vi "slow_control_alpha_06.vi"() -> ()   [LabVIEW 2018]
uses:
  <instrlib>/Lake Shore 335/Lake Shore 335.lvlib
  <instrlib>/CAEN PSM/CAEN PSM.lvlib
panel:
  in  "Cycles to execute":dbl=5.0 format="%#_13g"
  out "Moving average Det. P":dbl
  in  "N samples":i32=20
  in  "Allows tabs on \nfront panel":T1(tab)
  in  "Heater range":u16(ring) items=["Off", "Low (On)", "Medium", "High"]
  in  "Setpoint (°C)":dbl=-100.0 format="%.1f"
  in  "PID settings":cluster{"P":dbl, "I":dbl, "D":dbl}={"P"=50.0, "I"=20.0, "D"=120.0}
  in  "COM-port NI-box":refnum<visa-resource-name>
  in  "COM-port LakeShore":refnum<visa-resource-name>
  in  "ID Query":bool=TRUE
  in  "COM-port CAEN 1":refnum<visa-resource-name>
  in  "COM-port CAEN 2":refnum<visa-resource-name>
  in  "Sensor 2 Offset":dbl=1.0 format="%#_13g"
  in  "Sensor 2 Mult. Factor":dbl=25.0 format="%#_13g"
  in  "Sensor 1 Offset":dbl=0.44736 format="%#_13g"
  in  "Sensor 1 Mult. Factor":dbl=25.0 format="%#_13g"
  in  "Sensor 3 Offset":dbl=1.0 format="%#_13g"
  in  "Sensor 3 Mult. Factor":dbl=50.0 format="%#_13g"
  in  "Sensor 4 Offset":dbl=1.0 format="%#_13g"
  in  "Sensor 4 Mult. Factor":dbl=10.0 format="%#_13g"
  in  "Ignore Initialization Errors":bool caption="Ignore init. errors?"
  out "LakeShore status":bool
  out "NI-box status":bool
  out "CAEN 1 status":bool
  out "CAEN 2 status":bool
  out "Initialization status":bool
  out "Heater power (%)":cluster{timestamp[], dbl[]}[](graph)
  out "Flow (SLPM)":cluster{timestamp[], dbl[]}[](graph)
  out "Pressure":cluster{timestamp[], dbl[]}[](graph)
  out "Phase Diagram":cluster{"X":dbl, "Y":dbl}[](graph)
  in  "Temp. Channel selector":string(combo)="Average 15 to 20"
  out "Temperature":cluster{timestamp[], dbl[]}[](graph)
  in  "N samples":i32=30
  out "Average Flow (SLPM)":dbl caption="Average Flow (SLPM), of"
  in  "Pause?":bool
  out "Integrated Flow (SL)":dbl
  in  "Reset?":bool
  out "Coldhead":dbl
  out "Heater":dbl
  out "Temp. 1":dbl
  out "Temp. 2":dbl
  out "Temp. 3":dbl
  out "Temp. 4":dbl
  out "Temp. 5":dbl
  out "Temp. 6":dbl
  out "Temp. 7":dbl
  out "Temp. 8":dbl
  out "Temp. 9":dbl
  out "Temp. 10":dbl
  out "Temp. 11":dbl
  out "Temp. 12":dbl
  out "Temp. 13":dbl
  out "Temp. 14":dbl
  out "Temp. 15":dbl
  out "Temp. 16":dbl
  out "Temp. 17":dbl
  out "Temp. 18":dbl
  out "Temp. 19":dbl
  out "Temp. 20":dbl
  out "1 to 4":dbl[](array[numeric])
  out "5 to 8":dbl[](array[numeric])
  out "9 to 12":dbl[](array[numeric])
  out "13 to 16":dbl[](array[numeric])
  out "17 to 20":dbl[](array[numeric])
  out "Temp A":dbl
  out "Temp B":dbl
  in  "Temperature Channel selector":string(combo)="Average 15 to 20"
  out "Historical Large Phase Diagram":cluster{dbl[], dbl[]}[](graph)
  out "Large Phase Diagram":cluster{"X":dbl, "Y":dbl}[](graph)
  in  "Temperature Channel selector":string(combo)="Average 15 to 20"
  in  "Set to zero":bool
  out "Bottom gate":dbl(knob) scale=0.0..-3000.0
  out "Top gate":dbl(knob) scale=0.0..3000.0
  in  "Apply Voltage":bool
  in  "VSet (V)":dbl[](array[numeric])
  in  "IMax (uA)":dbl[](array[numeric])
  in  "VMax (V)":dbl[](array[numeric])
  out "Cathode":dbl(knob) scale=0.0..-5000.0
  out "Anode":dbl(knob) scale=0.0..4000.0
  out "PMT 2":dbl(knob) scale=0.0..1000.0
  out "PMT 1":dbl(knob) scale=1.0..1000.0
  out "Vmon (V)":dbl[](array[numeric])
  out "IMon (uA)":dbl[](array[numeric])
  out "Read V = 0":i32
  in  "Read V every N cycles":i16=120
  in  "Reset anode":bool
  in  "Kill every Y minutes":i32=10
  in  "Keep off for X seconds":i32=10
  out "?":bool
  out "Killed":bool
  out "Restarted":bool
  out "Anode times":dbl[](array[numeric]) format="%_12f"
  in  "Kill voltage":bool
  in  "stop":bool
  out "Voltages":dbl[](array[numeric])
  out "Started up?":bool
  out "TOBA appended":dbl[][](array[numeric])
  in  "Read T every N cycles":i32=2
  out "Time until next cycle":dbl format="%.3g"
  in  "Time per cycle (s)":i32=2 caption="Time Target (s)"
  in  "input cluster":errorcluster
  # "<- Proof of concept for New/Old T + New P"
  # "PMT 1"
  # "PMT 2"
  # "Anode"
  # "Cathode"
  # "Top gate"
  # "Bottom gate"
  # "Pressure correction settings"
  # "Connection settings"
  # "Lakeshore settings"
  # "Gain (P) (XX.X)"
  # "Reset (I) (XX.X)"
  # "Rate (D) (X.X%)"
  # "<- Change wiring,\nused for testing rn"
  # "Might need to split up NI-box com port.\nPreferable to task it with measuring T\nand P seperately.\nPerhaps need to set task per single channel."
  # "Alarm indicators"
  # "CAEN 1"
  # "Data"
  # "PMT 1"
  # "PMT 1"
  # "PMT 2"
  # "PMT 2"
  # "Anode"
  # "Anode"
  # "Cathode"
  # "Cathode"
  # "Top gate"
  # "Top gate"
  # "Bottom gate"
  # "Bottom gate"
  # "Settings"
  # "PMT 1"
  # "PMT 1"
  # "PMT 2"
  # "PMT 2"
  # "Anode"
  # "Anode"
  # "Cathode"
  # "Cathode"
  # "Top gate"
  # "Top gate"
  # "Bottom gate"
  # "Bottom gate"
  # "CAEN 2"
  # "PMT 1"
  # "PMT 2"
  # "Anode"
  # "seconds"
  # "Cathode"
  # "Needle gauges or other displays go here"
  # "Top gate"
  # "Bottom gate"
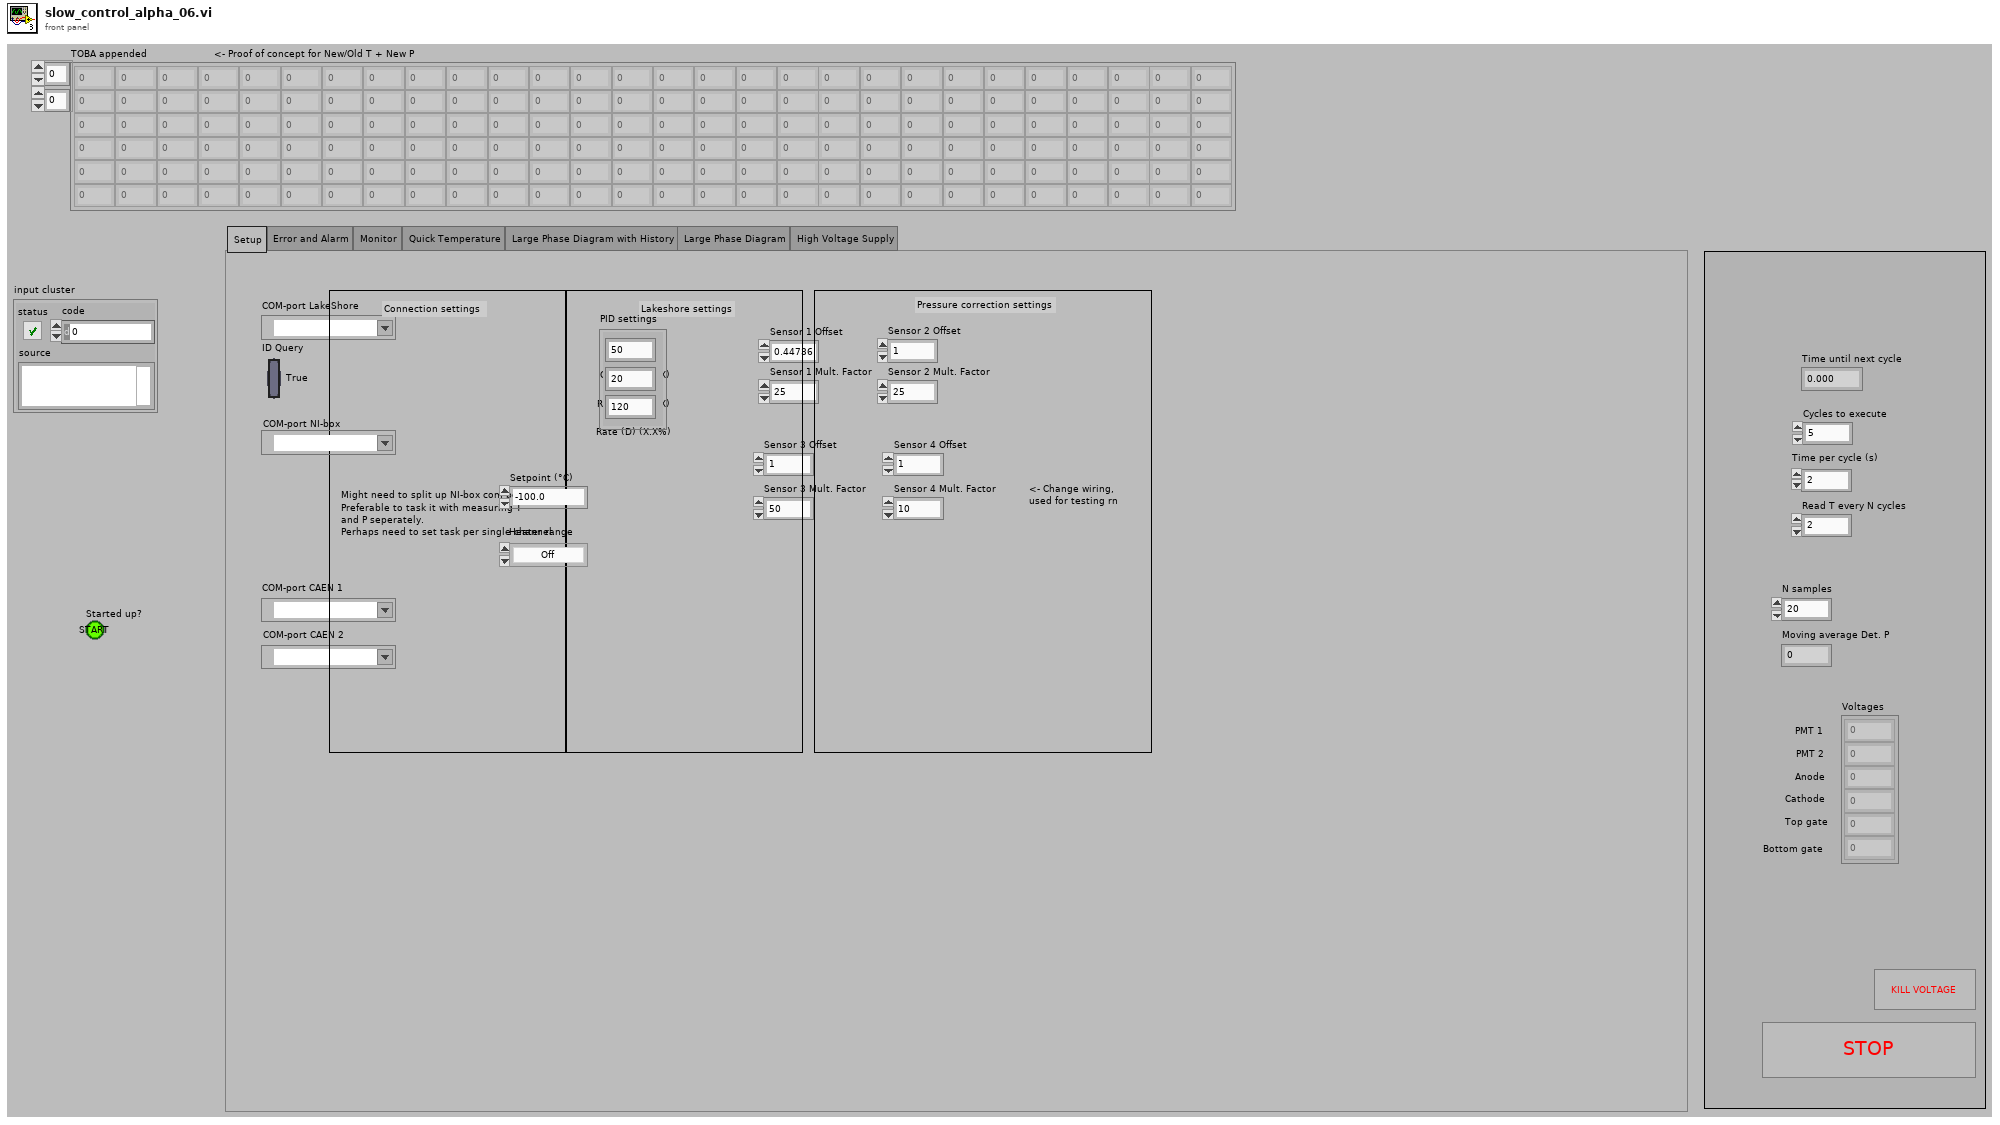
[diagram p1: front panel]
types:
  T1 = enum32{"Setup", "Error and Alarm", "Monitor", "Quick Temperature", "Large Phase Diagram with History", "Large Phase Diagram", "High Voltage Supply"}
  T2 = cluster{"Flow Control":u16, "Stop Bits":u16, "Data Bits":u16, "Parity":u16, "Baud Rate":u32}
  T3 = cluster{"VISA resource name out":refnum<visa-resource-name>, "error out":errorcluster}
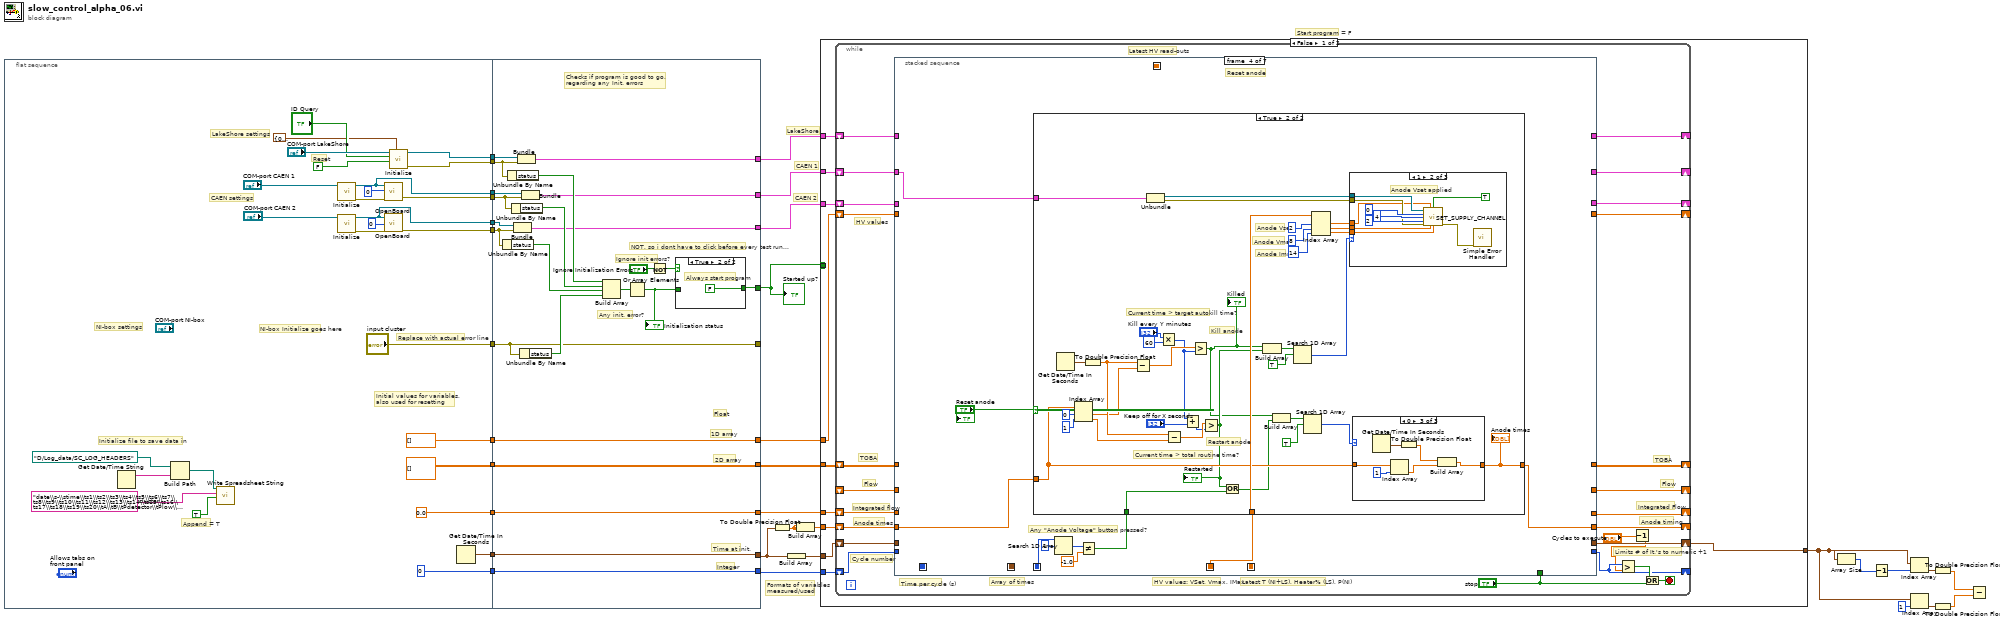
[diagram p0: block diagram]
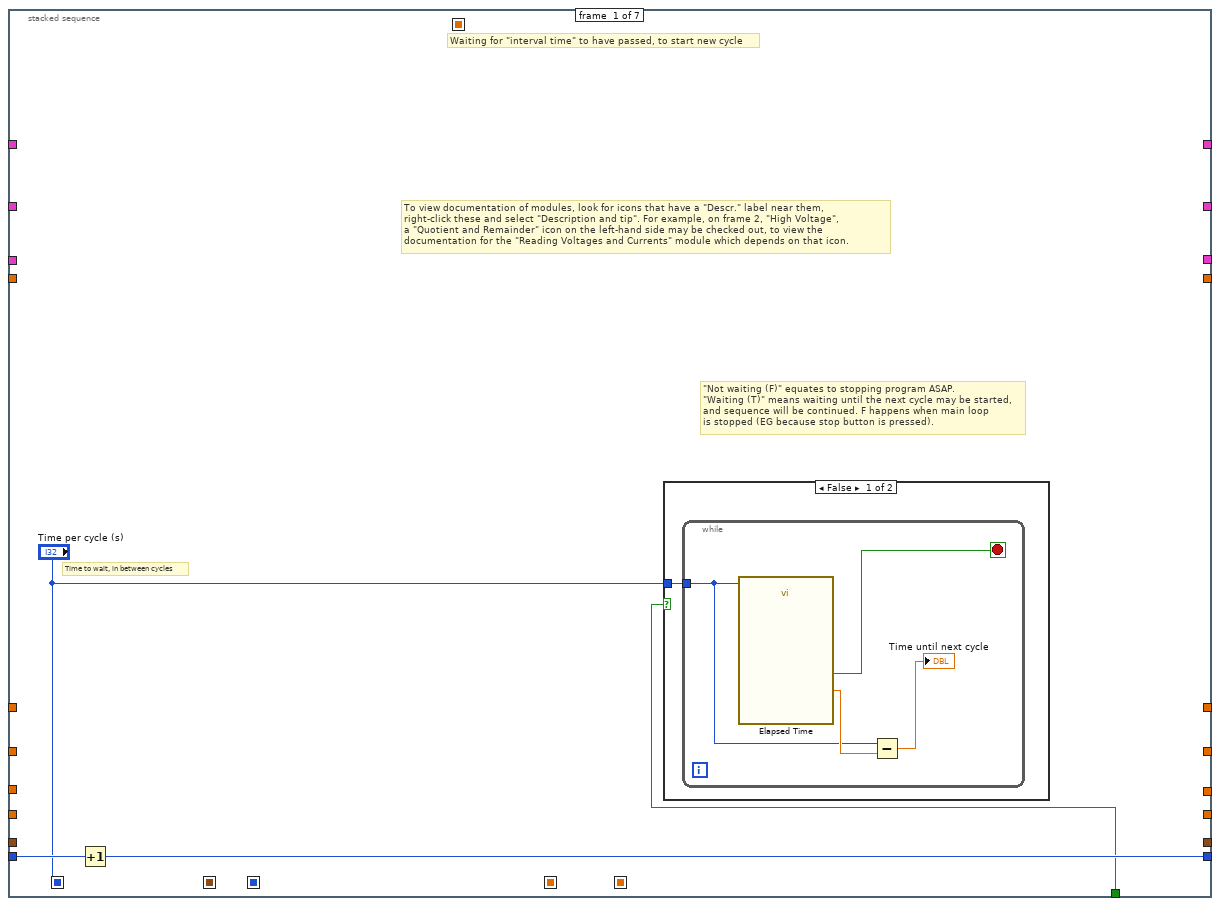
[diagram p2: hidden frame]
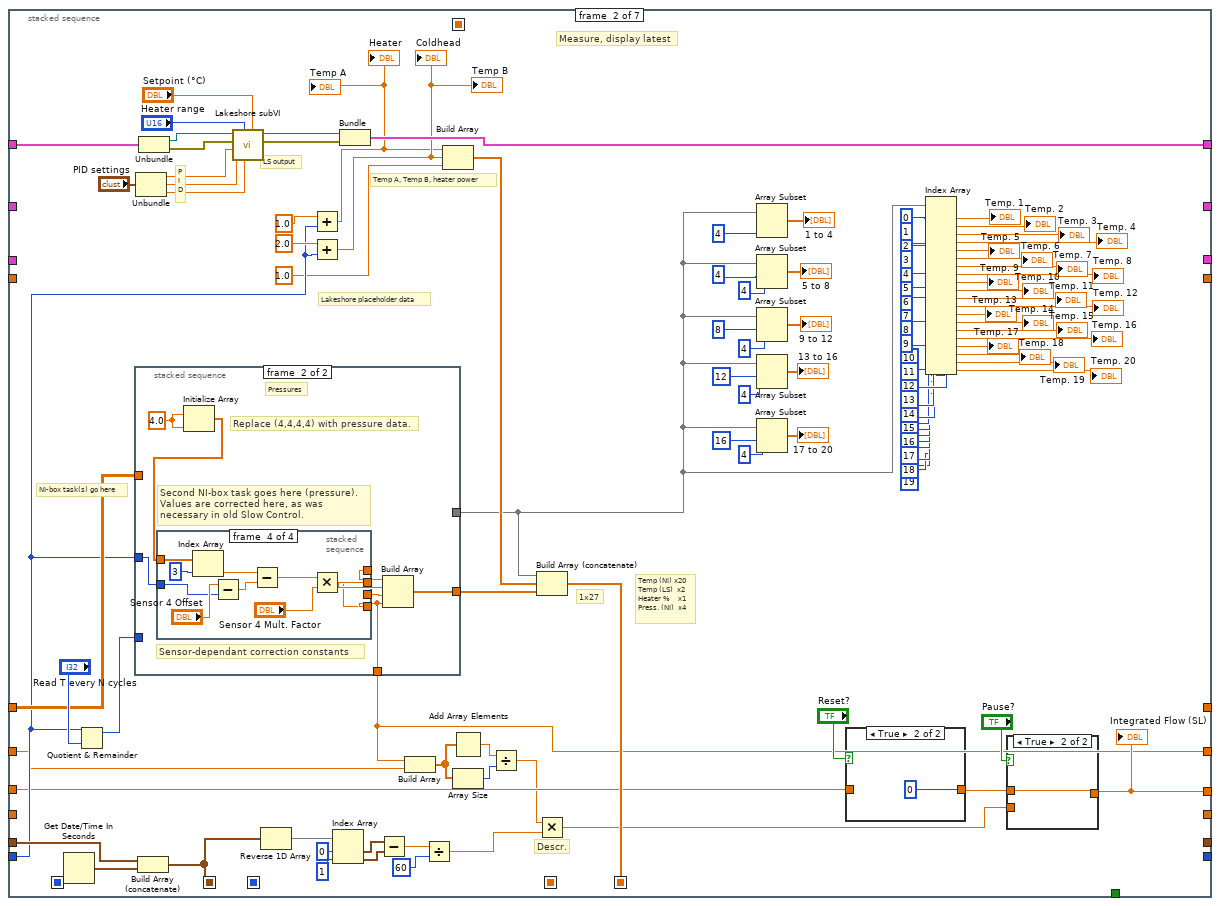
[diagram p4: hidden frame]
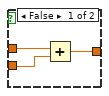
[diagram p6: hidden frame]
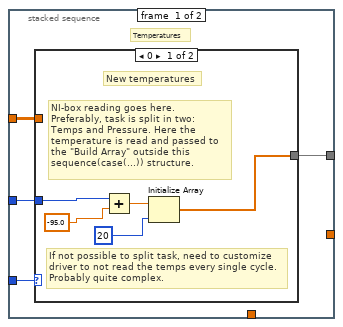
[diagram p7: hidden frame]
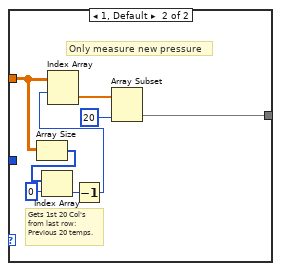
[diagram p8: hidden frame]
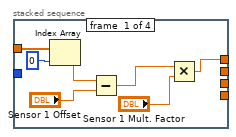
[diagram p9: hidden frame]
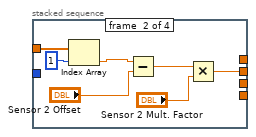
[diagram p10: hidden frame]
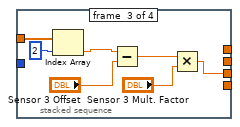
[diagram p11: hidden frame]
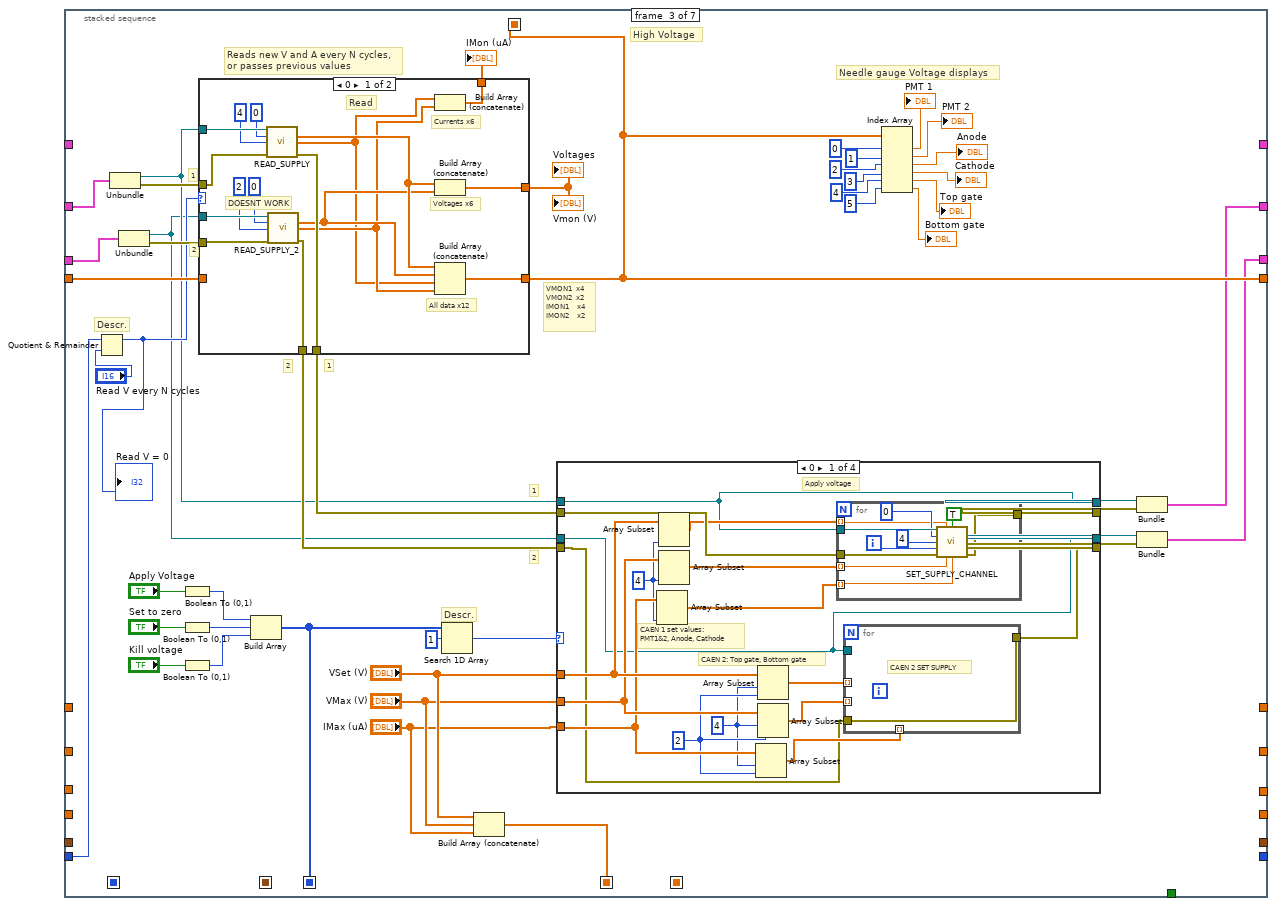
[diagram p12: hidden frame]
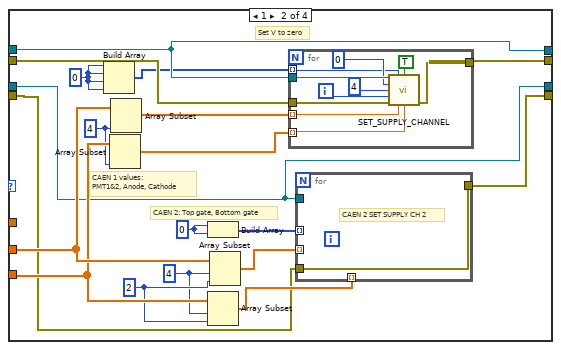
[diagram p13: hidden frame]
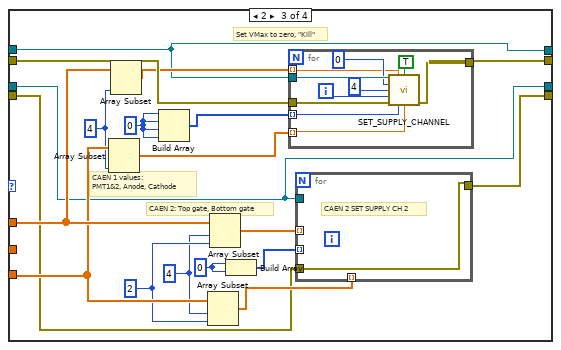
[diagram p14: hidden frame]
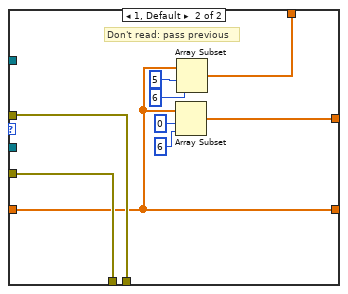
[diagram p16: hidden frame]
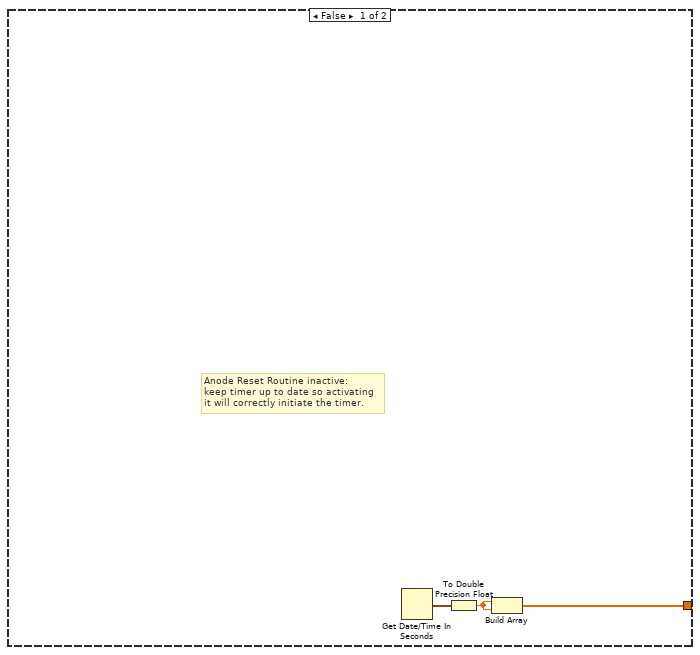
[diagram p17: hidden frame]
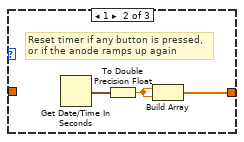
[diagram p19: hidden frame]
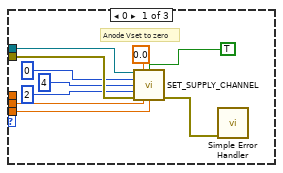
[diagram p20: hidden frame]
diagram:
  # "Start program = F"
  # "CAEN 2"
  # "CAEN 1"
  # "LakeShore"
  # "Formats of variables\nmeasured/used"
  n1 = flat-sequence {
    tunnel: [w56] -> w32
    tunnel: [w55] -> w31
    tunnel: [w51] -> w30
    tunnel: [w50] -> w29
    tunnel: ["input cluster"] -> w28
    tunnel: [0.0] -> w27
    tunnel: [dbl[] []] -> w26
    tunnel: [dbl[][] []] -> w25
    tunnel: [0] -> w24
    tunnel: [w38] -> w18
    tunnel: [w34] -> w8
    tunnel: [w33] -> w7
    tunnel: w32 -> [w72]
    tunnel: w31 -> [w71]
    tunnel: w30 -> [w69]
    tunnel: w29 -> [w68]
    tunnel: w28 -> [w73]
    tunnel: [w79] -> w5
    tunnel: [w77] -> w4
    tunnel: w27 -> [w77]
    tunnel: [w76] -> w23
    tunnel: w26 -> [w76]
    tunnel: [w75] -> w21
    tunnel: w25 -> [w75]
    tunnel: [w74] -> w22
    tunnel: w24 -> [w74]
    tunnel: [w73] -> _
    tunnel: [w70] -> w20
    tunnel: [w67] -> w19
    tunnel: [w64] -> w3
    tunnel: w18 -> [w64]
    tunnel: w8 -> [w62]
    tunnel: w7 -> [w61]
    tunnel: [w60] -> w6
    frame #0 {
      # "Append = T"
      # "Change to fit order of data in cluster"
      # "Initialize file to save data in"
      # "Initial values for variables,\nalso used for resetting"
      # "Replace with actual error line"
      # "NI-box Initialize goes here"
      # "NI-box settings"
      # "CAEN settings"
      # "Reset"
      # "LakeShore settings"
      n2 = Get Date/Time String() -> (date string=w41:string)  [unwired: 3 in, 1 out]
      n3 = Build Path(base path=path "D:/Log_data/SC_LOG_HEADERS", name or relative path=w41) -> (appended path=w44:path)
      n4 = call <vilib>:"Write Spreadsheet String.vi"("append to file? (new file:F)"=TRUE, "spreadsheet string"="date\\s-\\stime\\ts1\\ts2\\ts3\\ts4\\ts5\\ts6\\ts7\\ts8\\ts9\\ts10\\ts11\\ts12\\ts13\\ts14\\ts15\\ts16\\ts17\\ts18\\ts19\\ts20\\tA\\tB\\tPdetector\\tPlow\\tPhigh\\tFlow\\tHeater\\tSetpoint\\tCapacitance\\tTimestamp\\tInterval\\tLevel\\tV_PMT1\\tV_PMT2\\tV_Anode\\tV_cathode\\tI_PMT1\\tI_PMT2\\tI_Anode\\tI_cathode\\t\\r\\n", "file path (dialog if empty)"=w44) -> ()  [unwired: 7 in, 2 out]
      n5 = call <instrlib>:"Initialize.vi"("VISA resource name"="COM-port CAEN 1") -> ("error out"=w52:errorcluster, "VISA resource name out"=w51:refnum<visa-resource-name>)  [unwired: 9 in]
      n6 = call <instrlib>:"Initialize.vi"("VISA resource name"="COM-port CAEN 2") -> ("error out"=w35:errorcluster, "VISA resource name out"=w34:refnum<visa-resource-name>)  [unwired: 9 in]
      n7 = call <instrlib>:"OpenBoard.vi"("error in (no error)"=w52, "Board Address"=0, "VISA resource name"=w51) -> ("error out"=w50:errorcluster)  [unwired: 7 in, 1 out]
      n8 = call <instrlib>:"OpenBoard.vi"("error in (no error)"=w35, "Board Address"=u8 0, "VISA resource name"=w34) -> ("error out"=w33:errorcluster)  [unwired: 7 in, 1 out]
      n9 = call <instrlib>:"Initialize.vi"("Serial Configuration"=T2 {"Flow Control"=0, "Stop Bits"=10, "Data Bits"=7, "Parity"=1, "Baud Rate"=57600}, "Reset (True)"=FALSE ("Reset (LakeShore)"), "ID Query (True)"="ID Query", "VISA resource name"="COM-port LakeShore") -> ("error out"=w55:errorcluster, "VISA resource name out"=w56:refnum<visa-resource-name>)  [unwired: 6 in]
      n10 = Get Date/Time In Seconds() -> (seconds since 1Jan1904=w38:timestamp)
    }
    frame #1 {
      # "NOT, so i dont have to click before every test run..."
      # "Time at init."
      # "Integer"
      # "2D array"
      # "1D array"
      # "Float"
      # "Checks if program is good to go,\nregarding any Init. errors"
      # "Ignore init errors?"
      # "Any init. error?"
      n11 = Unbundle By Name(w61) -> ("status"=w63:bool)
      n12 = Unbundle By Name(w71) -> ("status"=w80:bool)
      n13 = Unbundle By Name(w68) -> ("status"=w82:bool)
      n14 = Bundle("VISA resource name out"=w62, "error out"=w61) -> (w60:T3)  [unwired: 1 in]
      n15 = Bundle("VISA resource name out"=w72, "error out"=w71) -> (w70:T3)  [unwired: 1 in]
      n16 = Unbundle By Name(w73) -> ("status"=w81:bool)
      n17 = Bundle("VISA resource name out"=w69, "error out"=w68) -> (w67:T3)  [unwired: 1 in]
      n18 = Build Array(w80, w82, w81, w63) -> (w83:bool[])
      n19 = Or Array Elements(Boolean array=w83) -> (logical OR=w78:bool)
      "Initialization status" <- w78
      n20 = Not(x="Ignore Initialization Errors") -> (.not. x?=w65:bool)
      n21 = case shown="True" w65 {
        tunnel: [w84 FALSE] -> w79
        tunnel: w78 -> [w84 _]
        frame False {
          # "Only start if no errors"
        }
        frame True {
          # "Always start program"
        }
      }
    }
  }
  n22 = To Double Precision Float(number=w3) -> (double precision float=w2:dbl)
  n23 = Build Array(w3) -> (w17:timestamp[])
  n24 = Build Array(w2, w2) -> (w1:dbl[])
  n25 = case shown="False" w5 {
    selector: w5 -> [_ w682]
    tunnel: [_ w682] -> _
    tunnel: w23 -> [w88 _]
    tunnel: w22 -> [w95 _]
    tunnel: w21 -> [w94 _]
    tunnel: w20 -> [w89 _]
    tunnel: w19 -> [w91 _]
    tunnel: w17 -> [w93 _]
    tunnel: [w92 timestamp[] []] -> w13
    tunnel: w6 -> [w90 _]
    tunnel: w4 -> [w87 _]
    tunnel: w1 -> [w86 _]
    frame False {
      n26 = while {
        shift-right: [w114] -> _
        shift-left: w95 -> [w120]
        shift-right: [w116] -> _
        shift-left: w94 -> [w105]
        shift-right: [w106] -> w92
        shift-left: w93 -> [w115]
        shift-right: [w108] -> _
        shift-left: w91 -> [w97]
        shift-right: [w110] -> _
        shift-left: w88 -> [w113]
        shift-right: [w107] -> _
        shift-left: w90 -> [w112]
        shift-right: [w109] -> _
        shift-left: w89 -> [w111]
        shift-right: [w104] -> _
        shift-left: w87 -> [w99]
        shift-right: [w101] -> _
        shift-left: _ -> [w100]
        shift-right: [w96] -> _
        shift-left: w86 -> [w98]
        stop <- w117 stop-if-true
        # "Anode timing"
        # "Anode times"
        # "Integrated flow"
        # "Flow"
        # "Flow"
        # "Integrated Flow"
        # "TOBA"
        # "Array of times"
        # "Latest HV read-outs"
        # "Time per cycle (s)"
        # "Cycle number"
        # "HV values: VSet, Vmax, IMax"
        # "HV values"
        # "TOBA"
        # "Latest T (NI+LS), Heater% (LS), P(NI)"
        # "Limits # of It.'s to numeric +1"
        n27 = stacked-sequence {
          seq-local: [_ w228 _ _ _ _ _] -> [_ _ _ _ w572 _ _]
          seq-local: [_ _ w294 _ _ _ _] -> [_ _ _ w460 _ _ _]
          seq-local: ["Time per cycle (s)" _ _ _ _ _ _] -> [_ _ _ _ _ _ _]
          seq-local: [_ _ w316 _ _ _ _] -> [_ _ _ _ _ _ _]
          seq-local: [_ w138 _ _ _ _ _] -> [_ _ _ _ w550 _ _]
          seq-local: [_ _ w293 _ _ _ _] -> [_ _ _ w465 _ _ _]
          tunnel: [w123 _ _ _ _ _ _] -> w114
          tunnel: "stop" -> [w122 _ _ _ _ _ _]
          tunnel: w120 -> [w124 w209 w331 _ _ _ _]
          tunnel: w105 -> [_ w229 _ _ w579 _ _]
          tunnel: [_ _ _ _ w571 _ _] -> w116
          tunnel: w115 -> [_ w215 _ _ _ _ _]
          tunnel: w97 -> [_ _ w338 w461 _ _ w678]
          tunnel: w113 -> [_ _ w336 _ _ _ _]
          tunnel: w112 -> [_ _ w335 _ _ _ w677]
          tunnel: w111 -> [_ w216 _ _ _ _ w675]
          tunnel: [_ w218 _ _ _ _ _] -> w109
          tunnel: [_ _ w316 _ _ _ _] -> w110
          tunnel: [_ _ w302 _ _ _ _] -> w108
          tunnel: [_ _ w299 _ _ _ _] -> w107
          tunnel: [_ _ _ _ w550 _ _] -> w106
          tunnel: w99 -> [_ w201 _ _ _ _ _]
          tunnel: [_ w202 _ _ _ _ _] -> w104
          tunnel: [_ w132 _ _ _ _ _] -> w101
          tunnel: w100 -> [_ w131 _ _ _ _ _]
          tunnel: w98 -> [_ _ _ w462 _ _ _]
          tunnel: [_ _ _ w458 _ _ _] -> w96
          frame #0 {
            # "To view documentation of modules, look for icons that have a \"Descr.\" label near them,\nright-click these and select \"Description and tip\". For example, on frame 2, \"High Voltage\",\na \"Quotient and Remainder\" icon on the left-hand side may be checked out, to view the\ndocumentation for the \"Reading Voltages and Currents\" module which depends on that icon."
            # "Time to wait, in between cycles"
            # "\"Not waiting (F)\" equates to stopping program ASAP.\n\"Waiting (T)\" means waiting until the next cycle may be started,\nand sequence will be continued. F happens when main loop \nis stopped (EG because stop button is pressed)."
            # "Waiting for \"interval time\" to have passed, to start new cycle"
            n28 = Increment(x=w124) -> (x+1=w123:i32)
            n29 = case shown="False" w122 {
              tunnel: "Time per cycle (s)" -> [w125 _]
              frame False {
                n30 = while {
                  tunnel: w125 -> [w127]
                  stop <- w129 stop-if-true
                  n31 = call "Elapsed Time"("Time Target (s)"=w127) -> ("Elapsed Time (s)"=w128:dbl, "Time has Elapsed"=w129:bool)  [unwired: 11 in, 6 out]
                  n32 = Subtract(x=w127, y=w128) -> (x-y=→"Time until next cycle":dbl)
                }
              }
              frame True {
              }
            }
          }
          frame #1 {
            # "1x27"
            # "Descr."
            # "LS output"
            # "Lakeshore placeholder data"
            # "Temp (NI) x20\nTemp (LS)  x2\nHeater %    x1\nPress. (NI)  x4"
            # "Temp A, Temp B, heater power"
            # "P\nI\nD"
            # "NI-box task(s) go here"
            # "Measure, display latest"
            n33 = Get Date/Time In Seconds() -> (seconds since 1Jan1904=w214:timestamp)
            n34 = Quotient & Remainder(x=w209, y="Read T every N cycles") -> (x-y*floor(x/y)=w230:i32)  [unwired: 1 out]
            n35 = stacked-sequence {
              tunnel: w230 -> [w241 _]
              tunnel: [w240 _] -> w136
              tunnel: [_ w259] -> w212
              tunnel: w229 -> [w239 _]
              tunnel: w209 -> [w238 w256]
              tunnel: [_ w255] -> w132
              frame #0 {
                # "Temperatures"
                n36 = case shown="0" w241 {
                  tunnel: w239 -> [_ w251]
                  tunnel: [w244 w247] -> w240
                  tunnel: w238 -> [w243 _]
                  frame 0 {
                    # "If not possible to split task, need to customize\ndriver to not read the temps every single cycle.\nProbably quite complex."
                    # "NI-box reading goes here.\nPreferably, task is split in two: \nTemps and Pressure. Here the \ntemperature is read and passed to \nthe \"Build Array\" outside this \nsequence(case(...)) structure."
                    # "New temperatures"
                    n37 = Add(x=w243, y=-95.0 ("element")) -> (x+y=w246:dbl)
                    n38 = Initialize Array(w246, 20) -> (w244:dbl[])
                  }
                  frame 1, Default {
                    # "Gets 1st 20 Col's\nfrom last row:\nPrevious 20 temps."
                    # "Only measure new pressure"
                    n39 = Array Size(array=w251) -> (size(s)=w253:i32[])
                    n40 = Index Array(array=w253, index=0) -> (element=w254:i32)
                    n41 = Decrement(x=w254) -> (x-1=w250:i32)
                    n42 = Index Array(array=w251, index (row)=w250) -> (element=w249:dbl[])  [unwired: 1 in]
                    n43 = Array Subset(array=w249, length=20) -> (w247:dbl[])  [unwired: 1 in]
                  }
                }
              }
              frame #1 {
                w258 = 4.0 ("element")
                # "Replace (4,4,4,4) with pressure data."
                # "Second NI-box task goes here (pressure).\nValues are corrected here, as was \nnecessary in old Slow Control."
                # "Sensor-dependant correction constants"
                # "Pressures"
                n44 = Initialize Array(w258, w258) -> (w257:dbl[])
                n45 = stacked-sequence {
                  tunnel: w257 -> [w264 w276 w283 w292]
                  tunnel: [w265 _ _ _] -> w262
                  tunnel: [_ w271 _ _] -> w261
                  tunnel: [_ _ w278 _] -> w260
                  tunnel: [_ _ _ w288] -> w255
                  tunnel: w256 -> [_ _ _ w284]
                  frame #0 {
                    n46 = Index Array(array=w264, index=0) -> (element=w263:dbl)
                    n47 = Subtract(x=w263, y="Sensor 1 Offset") -> (x-y=w267:dbl)
                    n48 = Multiply(x=w267, y="Sensor 1 Mult. Factor") -> (x*y=w265:dbl)
                  }
                  frame #1 {
                    n49 = Index Array(array=w276, index=1) -> (element=w270:dbl)
                    n50 = Subtract(x=w270, y="Sensor 2 Offset") -> (x-y=w273:dbl)
                    n51 = Multiply(x=w273, y="Sensor 2 Mult. Factor") -> (x*y=w271:dbl)
                  }
                  frame #2 {
                    n52 = Index Array(array=w283, index=2) -> (element=w277:dbl)
                    n53 = Subtract(x=w277, y="Sensor 3 Offset") -> (x-y=w280:dbl)
                    n54 = Multiply(x=w280, y="Sensor 3 Mult. Factor") -> (x*y=w278:dbl)
                  }
                  frame #3 {
                    n55 = Index Array(array=w292, index=3) -> (element=w287:dbl)
                    n56 = Subtract(x="Sensor 4 Offset", y=w284) -> (x-y=w286:dbl)
                    n57 = Subtract(x=w287, y=w286) -> (x-y=w290:dbl)
                    n58 = Multiply(x=w290, y="Sensor 4 Mult. Factor") -> (x*y=w288:dbl)
                  }
                }
                n59 = Build Array(w262, w261, w260, w255) -> (w259:dbl[])
              }
            }
            n60 = Unbundle("PID settings") -> ("P"=w224:dbl, "I"=w223:dbl, "D"=w222:dbl)
            n61 = Build Array (concatenate)(w215, w214) -> (w138:timestamp[])
            n62 = Unbundle(w216) -> ("VISA resource name out"=w226:refnum<visa-resource-name>, "error out"=w225:errorcluster)
            n63 = call "Lakeshore subVI.vi"("Setpoint"="Setpoint (°C)", "Rate (D) (X.X %)"=w222, "Range"="Heater range", "Reset (I) (XX.X)"=w223, "Gain (P) (XX.X)"=w224, "error in (no error)"=w225, "VISA resource name"=w226) -> ("error out"=w219:errorcluster, "VISA resource name out"=w220:refnum<visa-resource-name>)  [unwired: 3 out]
            n64 = Reverse 1D Array(array=w138) -> (reversed array=w143:timestamp[])
            n65 = Add(x=1.0, y=w209) -> (x+y=w184:dbl)
            "Temp A" <- w184
            "Heater" <- w184
            n66 = Add(x=2.0, y=w209) -> (x+y=w208:dbl)
            "Temp B" <- w208
            "Coldhead" <- w208
            n67 = Index Array(array=w143, index #1=0 ("index"), index #2=1 ("index")) -> (element #1=w140:timestamp, element #2=w139:timestamp)
            n68 = Bundle("VISA resource name out"=w220, "error out"=w219) -> (w218:T3)  [unwired: 1 in]
            n69 = Subtract(x=w140, y=w139) -> (x-y=w137:dbl)
            n70 = Build Array(w132, w131) -> (w133:dbl[])
            n71 = Divide(x=w137, y=60) -> (x/y=w205:dbl)
            n72 = Build Array(w184, w208, 1.0) -> (w213:dbl[])
            n73 = Add Array Elements(numeric array=w133) -> (sum=w134:dbl)
            n74 = Array Size(array=w133) -> (size(s)=w135:i32)
            n75 = Divide(x=w134, y=w135) -> (x/y=w130:dbl)
            n76 = Build Array (concatenate)(w136, w213, w212) -> (w228:dbl[])
            n77 = Multiply(x=w130, y=w205) -> (x*y=w200:dbl)
            n78 = Array Subset(array=w136, length=4) -> (→"1 to 4":dbl[])  [unwired: 1 in]
            n79 = Array Subset(array=w136, index=4, length=4 ("index")) -> (→"5 to 8":dbl[])
            n80 = Array Subset(array=w136, index=8, length=4 ("index")) -> (→"9 to 12":dbl[])
            n81 = Array Subset(array=w136, index=12, length=4 ("index")) -> (→"13 to 16":dbl[])
            n82 = Array Subset(array=w136, index=16, length=4 ("index")) -> (→"17 to 20":dbl[])
            n83 = case shown="True" "Reset?" {
              tunnel: w201 -> [w232 _]
              tunnel: [w232 0] -> w199
              frame False {
              }
              frame True {
              }
            }
            n84 = Index Array(array=w136, index #1=0, index #2=1, index #3=2, index #4=3, index #5=4, index #6=5, index #7=6, index #8=7, index #9=8, index #10=9, index #11=10, index #12=11, index #13=12, index #14=13, index #15=14, index #16=15, index #17=16, index #18=17, index #19=18, index #20=19) -> (element #1=→"Temp. 1":dbl, element #2=→"Temp. 2":dbl, element #3=→"Temp. 3":dbl, element #4=→"Temp. 4":dbl, element #5=→"Temp. 5":dbl, element #6=→"Temp. 6":dbl, element #7=→"Temp. 7":dbl, element #8=→"Temp. 8":dbl, element #9=→"Temp. 9":dbl, element #10=→"Temp. 10":dbl, element #11=→"Temp. 11":dbl, element #12=→"Temp. 12":dbl, element #13=→"Temp. 13":dbl, element #14=→"Temp. 14":dbl, element #15=→"Temp. 15":dbl, element #16=→"Temp. 16":dbl, element #17=→"Temp. 17":dbl, element #18=→"Temp. 18":dbl, element #19=→"Temp. 19":dbl, element #20=→"Temp. 20":dbl)
            n85 = case shown="True" "Pause?" {
              tunnel: w200 -> [w236 _]
              tunnel: w199 -> [w235 w237]
              tunnel: [w234 w237] -> w202
              frame False {
                n86 = Add(x=w235, y=w236) -> (x+y=w234:dbl)
              }
              frame True {
              }
            }
            "Integrated Flow (SL)" <- w202
          }
          frame #2 {
            # "2"
            # "1"
            # "Descr."
            # "Descr."
            # "VMON1  x4 \nVMON2  x2\nIMON1    x4\nIMON2    x2"
            # "Needle gauge Voltage displays"
            # "1"
            # "2"
            # "1"
            # "2"
            # "Reads new V and A every N cycles,\nor passes previous values"
            # "High Voltage"
            n87 = Quotient & Remainder(x=w331, y="Read V every N cycles") -> (x-y*floor(x/y)=w329:i32)  [unwired: 1 out]
            "Read V = 0" <- w329
            n88 = Unbundle(w338) -> ("VISA resource name out"=w305:refnum<visa-resource-name>, "error out"=w337:errorcluster)
            n89 = Unbundle(w335) -> ("VISA resource name out"=w304:refnum<visa-resource-name>, "error out"=w334:errorcluster)
            n90 = Boolean To (0,1)(Boolean="Apply Voltage") -> (0, 1=w312:i16)
            n91 = Boolean To (0,1)(Boolean="Set to zero") -> (0, 1=w311:i16)
            n92 = Boolean To (0,1)(Boolean="Kill voltage") -> (0, 1=w310:i16)
            n93 = case shown="0" w329 {
              tunnel: w305 -> [w448 _]
              tunnel: w337 -> [w447 w456]
              tunnel: w336 -> [_ w452]
              tunnel: w304 -> [w442 _]
              tunnel: w334 -> [w441 w457]
              tunnel: [w438 w457] -> w306
              tunnel: [w444 w456] -> w307
              tunnel: [w443 w452] -> w316
              tunnel: [w435 w453] -> w333
              tunnel: [w432 w449] -> w332
              frame 0 {
                # "DOESNT WORK"
                # "All data x12"
                # "Voltages x6"
                # "Currents x6"
                # "Read"
                n94 = call "READ_SUPPLY.vi"("VISA resource name"=w448, "Board address"=u8 0, "NChannels"=u8 4, "error in (no error)"=w447) -> ("VMon values (V)"=w437:dbl[], "IMon values (uA)"=w433:dbl[], "error out"=w444:errorcluster)  [unwired: 9 in]
                n95 = call "READ_SUPPLY_2.vi"("VISA resource name"=w442, "Board address"=u8 0, "NChannels"=u8 2, "error in (no error)"=w441) -> ("VMon values (V)"=w436:dbl[], "IMon values (uA)"=w434:dbl[], "error out"=w438:errorcluster)  [unwired: 9 in]
                n96 = Build Array (concatenate)(w433, w434) -> (w432:dbl[])
                n97 = Build Array (concatenate)(w437, w436) -> (w435:dbl[])
                n98 = Build Array (concatenate)(w437, w436, w433, w434) -> (w443:dbl[])
              }
              frame 1, Default {
                # "Don't read: pass previous"
                n99 = Array Subset(array=w452, index=0, length=6) -> (w453:dbl[])
                n100 = Array Subset(array=w452, index=5, length=6) -> (w449:dbl[])
              }
            }
            "Voltages" <- w333
            "Vmon (V)" <- w333
            "IMon (uA)" <- w332
            n101 = Build Array(w312, w311, w310) -> (w293:i16[])
            n102 = Search 1D Array(1D array=w293, element=i16 1) -> (index of element=w308:i32)  [unwired: 1 in]
            n103 = Build Array (concatenate)("VSet (V)", "VMax (V)", "IMax (uA)") -> (w294:dbl[])
            n104 = case shown="0" w308 {
              tunnel: w307 -> [w356 w386 w416 w428]
              tunnel: w306 -> [w342 w375 w405 w430]
              tunnel: w305 -> [w352 w383 w413 w431]
              tunnel: w304 -> [w340 w373 w403 w429]
              tunnel: [w353 w384 w414 w428] -> w298
              tunnel: [w352 w383 w413 w431] -> w303
              tunnel: [w339 w372 w402 w430] -> w300
              tunnel: [w340 w373 w403 w429] -> w301
              tunnel: "VSet (V)" -> [w350 _ w411 _]
              tunnel: "VMax (V)" -> [w349 w381 _ _]
              tunnel: "IMax (uA)" -> [w348 w380 w410 _]
              frame 0 {
                w341 = 4 ("length")
                w346 = 2 ("length")
                w347 = 4 ("length")
                # "CAEN 2: Top gate, Bottom gate"
                # "CAEN 1 set values:\nPMT1&2, Anode, Cathode"
                # "Apply voltage"
                n105 = Array Subset(array=w348, length=w347) -> (w351:dbl[])  [unwired: 1 in]
                n106 = Array Subset(array=w350, length=w347) -> (w355:dbl[])  [unwired: 1 in]
                n107 = Array Subset(array=w349, length=w347) -> (w354:dbl[])  [unwired: 1 in]
                n108 = Array Subset(array=w348, index=w341, length=w346) -> (w343:dbl[])
                n109 = Array Subset(array=w350, index=w341, length=w346) -> (w345:dbl[])
                n110 = Array Subset(array=w349, index=w341, length=w346) -> (w344:dbl[])
                n111 = for {
                  tunnel: w352 -> [w366]
                  tunnel: w356 -> [w365]
                  tunnel: w355 -> [w362] mode=indexing
                  tunnel: w354 -> [w360] mode=indexing
                  tunnel: w351 -> [w359] mode=indexing
                  tunnel: [w358] -> w353
                  i -> [w367]
                  n112 = call "SET_SUPPLY_CHANNEL.vi"("VISA resource name"=w366, "Voltage Level (0.0 V)"=w362, "Enable (OFF)"=TRUE, "Board address"=u8 0, "NChannels"=u8 4, "Channel (0)"=w367, "error in (no error)"=w365, "Voltage Max (0.0 V)"=w360, "Current Limit (0.00 uA)"=w359) -> ("error out"=w358:errorcluster)  [unwired: 6 in]
                }
                n113 = for {
                  tunnel: w340 -> [_]
                  tunnel: w342 -> [w357]
                  tunnel: w345 -> [_] mode=indexing
                  tunnel: w344 -> [_] mode=indexing
                  tunnel: w343 -> [_] mode=indexing
                  tunnel: [w357] -> w339
                  # "CAEN 2 SET SUPPLY"
                }
              }
              frame 1 {
                w368 = 0 ("length")
                w370 = 0 ("length")
                w374 = 4 ("length")
                w378 = 2 ("length")
                w379 = 4 ("length")
                # "CAEN 2: Top gate, Bottom gate"
                # "CAEN 1 values:\nPMT1&2, Anode, Cathode"
                # "Set V to zero"
                n114 = Build Array(w370, w370, w370, w370) -> (w371:i32[])
                n115 = Array Subset(array=w380, length=w379) -> (w382:dbl[])  [unwired: 1 in]
                n116 = Array Subset(array=w381, length=w379) -> (w385:dbl[])  [unwired: 1 in]
                n117 = Build Array(w368, w368) -> (w369:i32[])
                n118 = Array Subset(array=w380, index=w374, length=w378) -> (w376:dbl[])
                n119 = Array Subset(array=w381, index=w374, length=w378) -> (w377:dbl[])
                n120 = for {
                  tunnel: w383 -> [w396]
                  tunnel: w386 -> [w395]
                  tunnel: w371 -> [w392] mode=indexing
                  tunnel: w385 -> [w390] mode=indexing
                  tunnel: w382 -> [w389] mode=indexing
                  tunnel: [w388] -> w384
                  i -> [w397]
                  n121 = call "SET_SUPPLY_CHANNEL.vi"("VISA resource name"=w396, "Voltage Level (0.0 V)"=w392, "Enable (OFF)"=TRUE, "Board address"=u8 0, "NChannels"=u8 4, "Channel (0)"=w397, "error in (no error)"=w395, "Voltage Max (0.0 V)"=w390, "Current Limit (0.00 uA)"=w389) -> ("error out"=w388:errorcluster)  [unwired: 6 in]
                }
                n122 = for {
                  tunnel: w373 -> [_]
                  tunnel: w375 -> [w387]
                  tunnel: w369 -> [_] mode=indexing
                  tunnel: w377 -> [_] mode=indexing
                  tunnel: w376 -> [_] mode=indexing
                  tunnel: [w387] -> w372
                  # "CAEN 2 SET SUPPLY CH 2"
                }
              }
              frame 2 {
                w399 = 0 ("length")
                w401 = 0 ("length")
                w404 = 4 ("length")
                w408 = 2 ("length")
                w409 = 4 ("length")
                # "CAEN 2: Top gate, Bottom gate"
                # "CAEN 1 values:\nPMT1&2, Anode, Cathode"
                # "Set VMax to zero, \"Kill\""
                n123 = Array Subset(array=w410, length=w409) -> (w412:dbl[])  [unwired: 1 in]
                n124 = Array Subset(array=w411, length=w409) -> (w415:dbl[])  [unwired: 1 in]
                n125 = Build Array(w401, w401, w401, w401) -> (w400:i32[])
                n126 = Array Subset(array=w410, index=w404, length=w408) -> (w406:dbl[])
                n127 = Array Subset(array=w411, index=w404, length=w408) -> (w407:dbl[])
                n128 = Build Array(w399, w399) -> (w398:i32[])
                n129 = for {
                  tunnel: w413 -> [w426]
                  tunnel: w416 -> [w425]
                  tunnel: w415 -> [w422] mode=indexing
                  tunnel: w400 -> [w420] mode=indexing
                  tunnel: w412 -> [w419] mode=indexing
                  tunnel: [w418] -> w414
                  i -> [w427]
                  n130 = call "SET_SUPPLY_CHANNEL.vi"("VISA resource name"=w426, "Voltage Level (0.0 V)"=w422, "Enable (OFF)"=TRUE, "Board address"=u8 0, "NChannels"=u8 4, "Channel (0)"=w427, "error in (no error)"=w425, "Voltage Max (0.0 V)"=w420, "Current Limit (0.00 uA)"=w419) -> ("error out"=w418:errorcluster)  [unwired: 6 in]
                }
                n131 = for {
                  tunnel: w403 -> [_]
                  tunnel: w405 -> [w417]
                  tunnel: w407 -> [_] mode=indexing
                  tunnel: w398 -> [_] mode=indexing
                  tunnel: w406 -> [_] mode=indexing
                  tunnel: [w417] -> w402
                  # "CAEN 2 SET SUPPLY CH 2"
                }
              }
              frame 3, Default {
                # "\"Executes\" if none of the three buttons have been clicked"
                # "Do nothing"
              }
            }
            n132 = Index Array(array=w316, index #1=0 ("index"), index #2=1 ("index"), index #3=2 ("index"), index #4=3 ("index"), index #5=4 ("index"), index #6=5 ("index")) -> (element #1=→"PMT 1":dbl, element #2=→"PMT 2":dbl, element #3=→"Anode":dbl, element #4=→"Cathode":dbl, element #5=→"Top gate":dbl, element #6=→"Bottom gate":dbl)
            n133 = Bundle("VISA resource name out"=w303, "error out"=w298) -> (w302:T3)  [unwired: 1 in]
            n134 = Bundle("VISA resource name out"=w301, "error out"=w300) -> (w299:T3)  [unwired: 1 in]
          }
          frame #3 {
            # "Any \"Anode Voltage\" button pressed?"
            # "Reset anode"
            n135 = Search 1D Array(1D array=w465, element=i16 1) -> (index of element=w466:i32)  [unwired: 1 in]
            n136 = Not Equal?(x=w466, y=-1.0) -> (x != y?=w459:bool)
            n137 = case shown="True" "Reset anode" {
              tunnel: w462 -> [_ w488]
              tunnel: w461 -> [_ w502]
              tunnel: w460 -> [_ w499]
              tunnel: w459 -> [_ w491]
              tunnel: [w468 w490] -> w458
              frame False {
                # "Anode Reset Routine inactive:\nkeep timer up to date so activating\nit will correctly initiate the timer."
                n138 = Get Date/Time In Seconds() -> (seconds since 1Jan1904=w470:timestamp)
                n139 = To Double Precision Float(number=w470) -> (double precision float=w469:dbl)
                n140 = Build Array(w469, w469) -> (w468:dbl[])
              }
              frame True {
                # "Anode Imax"
                # "Anode Vmax"
                # "Anode Vset"
                # "Current time > total routine time?"
                # "Restart anode"
                # "Kill anode"
                # "Current time > target autokill time?"
                n141 = Get Date/Time In Seconds() -> (seconds since 1Jan1904=w504:timestamp)
                n142 = Index Array(array=w488, index #1=0 ("index"), index #2=1 ("index")) -> (element #1=w482:dbl, element #2=w484:dbl)
                n143 = To Double Precision Float(number=w504) -> (double precision float=w483:dbl)
                n144 = Subtract(x=w483, y=w482) -> (x-y=w481:dbl)
                n145 = Unbundle(w502) -> ("VISA resource name out"=w501:refnum<visa-resource-name>, "error out"=w500:errorcluster)
                n146 = Multiply(x="Kill every Y minutes", y=60) -> (x*y=w480:i32)
                n147 = Subtract(x=w483, y=w484) -> (x-y=w472:dbl)
                n148 = Add(x=w480, y="Keep off for X seconds") -> (x+y=w471:i32)
                n149 = Greater?(x=w481, y=w480) -> (0:w474:bool)
                "Killed" <- w474
                n150 = Greater?(x=w472, y=w471) -> (0:w475:bool)
                "Restarted" <- w475
                n151 = Or(x=w475, y=w491) -> (x .or. y?=w478:bool)
                n152 = Build Array(w474, w475) -> (w493:bool[])
                n153 = Build Array(w474, w478) -> (w479:bool[])
                n154 = Search 1D Array(1D array=w493, element=TRUE) -> (index of element=w492:i32)  [unwired: 1 in]
                n155 = Search 1D Array(1D array=w479, element=TRUE) -> (index of element=w476:i32)  [unwired: 1 in]
                n156 = Index Array(array=w499, index #1=2 ("index"), index #2=8 ("index"), index #3=14 ("index")) -> (element #1=w496:dbl, element #2=w494:dbl, element #3=w495:dbl)
                n157 = case shown="1" w492 {
                  tunnel: w496 -> [_ w529 _]
                  tunnel: w494 -> [w517 w528 _]
                  tunnel: w495 -> [w519 w527 _]
                  tunnel: w501 -> [w525 w532 _]
                  tunnel: w500 -> [w524 w531 _]
                  frame 0 {
                    # "Anode Vset to zero"
                    n158 = call "SET_SUPPLY_CHANNEL.vi"("VISA resource name"=w525, "Voltage Level (0.0 V)"=0.0, "Enable (OFF)"=TRUE, "Board address"=u8 0, "NChannels"=u8 4, "Channel (0)"=u8 2, "error in (no error)"=w524, "Voltage Max (0.0 V)"=w517, "Current Limit (0.00 uA)"=w519) -> ("error out"=w518:errorcluster)  [unwired: 6 in]
                    n159 = call <vilib>:"Simple Error Handler.vi"("error in (no error)"=w518) -> ()  [unwired: 4 in, 5 out]
                  }
                  frame 1 {
                    # "Anode Vset applied"
                    n160 = call "SET_SUPPLY_CHANNEL.vi"("VISA resource name"=w532, "Voltage Level (0.0 V)"=w529, "Enable (OFF)"=TRUE, "Board address"=u8 0, "NChannels"=u8 4, "Channel (0)"=u8 2, "error in (no error)"=w531, "Voltage Max (0.0 V)"=w528, "Current Limit (0.00 uA)"=w527) -> ("error out"=w526:errorcluster)  [unwired: 6 in]
                    n161 = call <vilib>:"Simple Error Handler.vi"("error in (no error)"=w526) -> ()  [unwired: 4 in, 5 out]
                  }
                  frame 2, Default {
                    # "Do nothing"
                  }
                }
                n162 = case shown="0" w476 {
                  tunnel: [w506 w507 w510] -> w490
                  tunnel: w488 -> [w506 _ w514]
                  frame 2, Default {
                    # "Time difference keeps \nincrementing for now"
                  }
                  frame 1 {
                    # "Reset timer if any button is pressed,\nor if the anode ramps up again"
                    n163 = Get Date/Time In Seconds() -> (seconds since 1Jan1904=w509:timestamp)
                    n164 = To Double Precision Float(number=w509) -> (double precision float=w508:dbl)
                    n165 = Build Array(w508, w508) -> (w507:dbl[])
                  }
                  frame 0 {
                    n166 = Get Date/Time In Seconds() -> (seconds since 1Jan1904=w513:timestamp)
                    n167 = Index Array(array=w514, index=1) -> (element=w511:dbl)
                    n168 = To Double Precision Float(number=w513) -> (double precision float=w512:dbl)
                    n169 = Build Array(w512, w511) -> (w510:dbl[])
                  }
                }
                "Anode times" <- w490
              }
            }
            "?" <- "Reset anode"
          }
          frame #4 {
            # "Moving averages"
            # "Plots heater power vs. t"
            # "Historic graphs: Phase, Pressure, Flow, Heater, Temperature"
            # "Plots flow vs. t"
            # "Plots three pressures vs. t in one graph"
            # "Non-historic Temperature + Det. Pressure"
            # "Det., Low, High, Flow, Heater\nentire columns"
            # "Latest readings (NI, LS)"
            # "Single Temp.'s"
            # "Single Temp.'s"
            # "Updated TOBA"
            # "Descr."
            # "Latest Detector Pressure"
            # "Plots individual lists of Temp. vs. t"
            # "Plots and moving averages"
            n170 = Build Array (concatenate)(w579, w572) -> (w571:dbl[][])
            "TOBA appended" <- w571
            n171 = case shown="\"Channel 17\", Default" "Temperature Channel selector" {
              tunnel: w571 -> [w587 w590 w593 w596 w599 w602 w605 w608]
              tunnel: [w586 w589 w592 w595 w598 w601 w604 w607] -> w568
              frame "Channel 15" {
                n172 = Index Array(array=w587, index (col)=14) -> (element=w586:dbl[])  [unwired: 1 in]
              }
              frame "Channel 16" {
                n173 = Index Array(array=w590, index (col)=15) -> (element=w589:dbl[])  [unwired: 1 in]
              }
              frame "Channel 17", Default {
                n174 = Index Array(array=w593, index (col)=16) -> (element=w592:dbl[])  [unwired: 1 in]
              }
              frame "Channel 18" {
                n175 = Index Array(array=w596, index (col)=17) -> (element=w595:dbl[])  [unwired: 1 in]
              }
              frame "Channel 19" {
                n176 = Index Array(array=w599, index (col)=18) -> (element=w598:dbl[])  [unwired: 1 in]
              }
              frame "Channel 20" {
                n177 = Index Array(array=w602, index (col)=19) -> (element=w601:dbl[])  [unwired: 1 in]
              }
              frame "Channel A" {
                n178 = Index Array(array=w605, index (col)=20) -> (element=w604:dbl[])  [unwired: 1 in]
              }
              frame "Channel B" {
                n179 = Index Array(array=w608, index (col)=21) -> (element=w607:dbl[])  [unwired: 1 in]
              }
            }
            n180 = case shown="\"Average 15 to 20\", Default" "Temp. Channel selector" {
              tunnel: w572 -> [w642 w644 w647 w650 w653 w656 w659 w662 w669]
              tunnel: [w640 w643 w646 w649 w652 w655 w658 w661 w664] -> w582
              frame "Channel 15" {
                n181 = Index Array(array=w642, index=14) -> (element=w640:dbl)
              }
              frame "Channel 16" {
                n182 = Index Array(array=w644, index=15) -> (element=w643:dbl)
              }
              frame "Channel 17" {
                n183 = Index Array(array=w647, index=16) -> (element=w646:dbl)
              }
              frame "Channel 18" {
                n184 = Index Array(array=w650, index=17) -> (element=w649:dbl)
              }
              frame "Channel 19" {
                n185 = Index Array(array=w653, index=18) -> (element=w652:dbl)
              }
              frame "Channel 20" {
                n186 = Index Array(array=w656, index=19) -> (element=w655:dbl)
              }
              frame "Channel A" {
                n187 = Index Array(array=w659, index=20) -> (element=w658:dbl)
              }
              frame "Channel B" {
                n188 = Index Array(array=w662, index=21) -> (element=w661:dbl)
              }
              frame "Average 15 to 20", Default {
                w665 = 6 ("length")
                n189 = Array Subset(array=w669, index=14, length=w665) -> (w667:dbl[])
                n190 = Add Array Elements(numeric array=w667) -> (sum=w666:dbl)
                n191 = Divide(x=w666, y=w665) -> (x/y=w664:dbl)
              }
            }
            n192 = for {
              N: 22 -> [_]
              tunnel: w550 -> [w674]
              tunnel: [w673] -> w584 mode=indexing
              tunnel: w571 -> [w672]
              i -> [w671]
              n193 = Index Array(array=w672, index (col)=w671) -> (element=w670:dbl[])  [unwired: 1 in]
              n194 = Bundle(w674, w670) -> (w673:cluster{timestamp[], dbl[]})  [unwired: 1 in]
            }
            "Temperature" <- w584
            n195 = Index Array(array=w571, index (col) #1=23 ("disabled index (col)"), index (col) #2=24 ("index (col)"), index (col) #3=25 ("index (col)"), index (col) #4=26 ("index (col)"), index (col) #5=22 ("index (col)")) -> (element #1=w549:dbl[], element #2=w563:dbl[], element #3=w562:dbl[], element #4=w542:dbl[], element #5=w553:dbl[])  [unwired: 5 in]
            n196 = Bundle(w568, w549) -> (w567:cluster{dbl[], dbl[]})  [unwired: 1 in]
            n197 = Index Array(array=w572, index=23) -> (element=w573:dbl)
            n198 = Bundle(w550, w553) -> (w552:cluster{timestamp[], dbl[]})  [unwired: 1 in]
            n199 = Bundle(w550, w549) -> (w561:cluster{timestamp[], dbl[]})  [unwired: 1 in]
            n200 = Bundle(w550, w563) -> (w560:cluster{timestamp[], dbl[]})  [unwired: 1 in]
            n201 = Bundle(w550, w562) -> (w559:cluster{timestamp[], dbl[]})  [unwired: 1 in]
            n202 = Bundle(w550, w542) -> (w556:cluster{timestamp[], dbl[]})  [unwired: 1 in]
            n203 = Bundle(w582, w573) -> (w581:cluster{dbl, dbl})  [unwired: 1 in]
            n204 = Build Array(w567) -> (→"Historical Large Phase Diagram":cluster{dbl[], dbl[]}[])
            n205 = Build Array(w581) -> (→"Phase Diagram":cluster{dbl, dbl}[])
            n206 = Build Array(w556) -> (→"Flow (SLPM)":cluster{timestamp[], dbl[]}[])
            n207 = Build Array(w552) -> (→"Heater power (%)":cluster{timestamp[], dbl[]}[])
            n208 = Build Array(w561, w560, w559) -> (→"Pressure":cluster{timestamp[], dbl[]}[])
            n209 = case shown="\"Average 15 to 20\", Default" "Temperature Channel selector" {
              tunnel: w572 -> [w612 w614 w617 w620 w623 w626 w629 w632 w639]
              tunnel: [w610 w613 w616 w619 w622 w625 w628 w631 w634] -> w577
              frame "Channel 15" {
                n210 = Index Array(array=w612, index=14) -> (element=w610:dbl)
              }
              frame "Channel 16" {
                n211 = Index Array(array=w614, index=15) -> (element=w613:dbl)
              }
              frame "Channel 17" {
                n212 = Index Array(array=w617, index=16) -> (element=w616:dbl)
              }
              frame "Channel 18" {
                n213 = Index Array(array=w620, index=17) -> (element=w619:dbl)
              }
              frame "Channel 19" {
                n214 = Index Array(array=w623, index=18) -> (element=w622:dbl)
              }
              frame "Channel 20" {
                n215 = Index Array(array=w626, index=19) -> (element=w625:dbl)
              }
              frame "Channel A" {
                n216 = Index Array(array=w629, index=20) -> (element=w628:dbl)
              }
              frame "Channel B" {
                n217 = Index Array(array=w632, index=21) -> (element=w631:dbl)
              }
              frame "Average 15 to 20", Default {
                w635 = 6 ("length")
                n218 = Array Subset(array=w639, index=14, length=w635) -> (w637:dbl[])
                n219 = Add Array Elements(numeric array=w637) -> (sum=w636:dbl)
                n220 = Divide(x=w636, y=w635) -> (x/y=w634:dbl)
              }
            }
            n221 = Reverse 1D Array(array=w549) -> (reversed array=w548:dbl[])
            n222 = Reverse 1D Array(array=w542) -> (reversed array=w544:dbl[])
            n223 = Array Subset(array=w548, length="N samples") -> (w537:dbl[])  [unwired: 1 in]
            n224 = Array Subset(array=w544, length="N samples") -> (w539:dbl[])  [unwired: 1 in]
            n225 = Array Size(array=w539) -> (size(s)=w538:i32)
            n226 = Array Size(array=w537) -> (size(s)=w536:i32)
            n227 = Add Array Elements(numeric array=w539) -> (sum=w543:dbl)
            n228 = Add Array Elements(numeric array=w537) -> (sum=w547:dbl)
            n229 = Divide(x=w543, y=w538) -> (x/y=→"Average Flow (SLPM)":dbl)
            n230 = Divide(x=w547, y=w536) -> (x/y=→"Moving average Det. P":dbl)
            n231 = Bundle(w577, w573) -> (w578:cluster{dbl, dbl})  [unwired: 1 in]
            n232 = Build Array(w578) -> (→"Large Phase Diagram":cluster{dbl, dbl}[])
          }
          frame #5 {
            # "Remaining displays"
          }
          frame #6 {
            # "Checking alarms"
            n233 = Unbundle By Name(w677) -> ("error out.status"=→"CAEN 2 status":bool)
            n234 = Unbundle By Name(w678) -> ("error out.status"=→"CAEN 1 status":bool)
            n235 = Unbundle By Name(w675) -> ("error out.status"=→"LakeShore status":bool)
          }
        }
        n236 = Decrement(x="Cycles to execute") -> (x-1=w102:dbl)
        n237 = Greater?(x=w114, y=w102) -> (0:w119:bool)
        n238 = Or(x=w119, y="stop") -> (x .or. y?=w117:bool)
      }
    }
    frame True {
    }
  }
  n239 = Array Size(array=w13) -> (size(s)=w16:i32)
  n240 = Decrement(x=w16) -> (x-1=w15:i32)
  n241 = Index Array(array=w13, index=w15) -> (element=w14:timestamp)
  n242 = Index Array(array=w13, index=1) -> (element=w11:timestamp)
  n243 = To Double Precision Float(number=w14) -> (double precision float=w10:dbl)
  n244 = To Double Precision Float(number=w11) -> (double precision float=w9:dbl)
  n245 = Subtract(x=w10, y=w9) -> ()  [unwired: 1 out]
  "Started up?" <- w5
